vi "AnalogWaveformProbe_I16.vi"(1 "Waveform":waveform(i16)={"t0"=timestamp(0 s since 1904-01-01), "dt"=0.0, "Y"=[]}) -> (0 "Stop if?":bool)   [LabVIEW 2017]
doc: "Displays a graph of the analog data; a table with a time stamp that specifies when the probe received the data, the x value, and the time; and a table that displays the attributes of the waveform data type."
uses:
  <vilib>/Utility/error.llb/ErrWarn.ctl
panel:
  in  "x":string="x"
  in  "t":string="t"
  in  "Tab Control":T1(tab)
  out "Timestamp":timestamp format="%<%X\n%x>T"
  out "Waveform Graph":waveform(i16)(graph) caption="Waveform Graph 2"
  in  "warn icon":T2
  in  "warning msg":string="Table data truncated to\nlimit memory usage."
  out "Start t":timestamp format="%<%X\n%x>T"
  out "Data":string[][](table)
  out "Attributes":variant
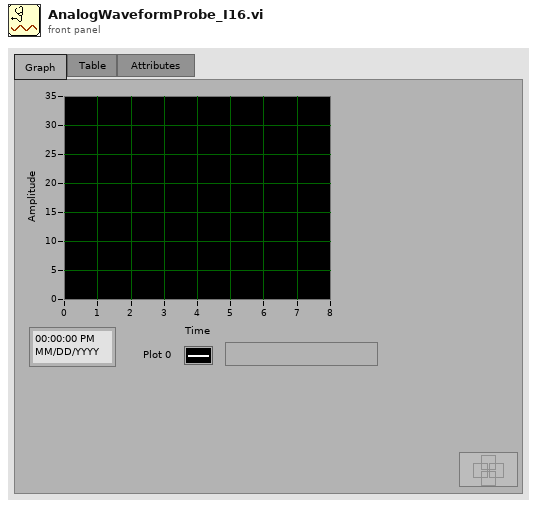
[diagram p1: front panel]
types:
  T1 = enum32{"Graph   ", "Table   ", "Attributes     "}
  T2 = typedef "ErrWarn.ctl" = bool
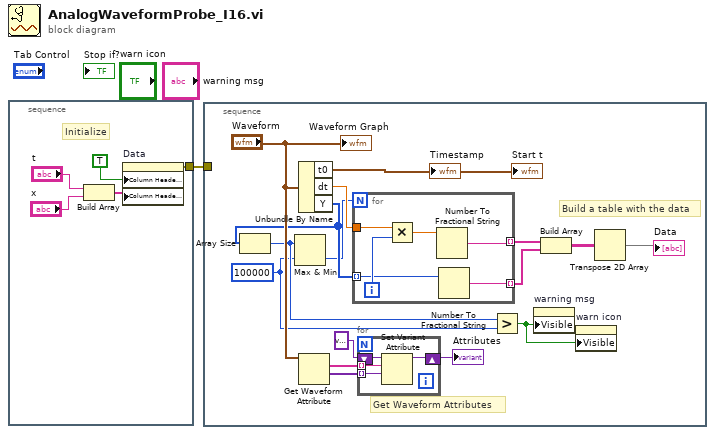
[diagram p0: block diagram]
diagram:
  n1 = stacked-sequence {
    tunnel: [w2] -> w1
    frame #0 {
      # "Initialize"
      n2 = Build Array("t", "x") -> (w4:string[])
      n3 = property on="Data" class="Tbl (strict)"("Column Headers Visible"=TRUE, "Column Header Strings[]"=w4) -> (error out=w2:errorcluster)  [unwired: 2 in, 1 out]
    }
  }
  n4 = stacked-sequence {
    tunnel: w1 -> [_]
    frame #0 {
      w8 = 100000
      # "Get Waveform Attributes"
      # "Build a table with the data"
      n5 = Unbundle By Name("Waveform") -> ("t0"=→"Timestamp" →"Start t":timestamp, "dt"=w22:dbl, "Y"=w11:i16[])
      n6 = Array Size(array=w11) -> (size(s)=w9:i32)
      n7 = Max & Min(x=w9, y=w8) -> (min(x,y)=w10:i32)  [unwired: 1 out]
      n8 = Get Waveform Attribute(7:"Waveform") -> (1:w14:variant[], 2:w15:string[])  [unwired: 3 in, 2 out]
      n9 = for {
        N: w10 -> [_]
        tunnel: [w30] -> w19 mode=indexing
        tunnel: w11 -> [w29] mode=indexing
        tunnel: w22 -> [w32]
        tunnel: [w27] -> w18 mode=indexing
        i -> [w31]
        n10 = Multiply(x=w32, y=w31) -> (x*y=w28:dbl)
        n11 = Number To Fractional String(number=w28) -> (F-format string=w27:string)  [unwired: 3 in]
        n12 = Number To Fractional String(number=w29) -> (F-format string=w30:string)  [unwired: 3 in]
      }
      n13 = for {
        tunnel: w15 -> [w25] mode=indexing
        tunnel: w14 -> [w26] mode=indexing
        shift-right: [w23] -> w12
        shift-left: variant ("variant") -> [w24]
        n14 = Set Variant Attribute(Variant=w24, name=w25, value=w26) -> (Variant out=w23:variant)  [unwired: 1 in, 2 out]
      }
      "Attributes" <- w12
      n15 = Greater?(x=w9, y=w8) -> (0:w7:bool)
      n16 = property on="warning msg" class="Str"("Visible"=w7) -> ()  [unwired: 2 in, 2 out]
      n17 = Build Array(w18, w19) -> (w21:string[][])
      n18 = property on="warn icon" class="Bool"("Visible"=w7) -> ()  [unwired: 2 in, 2 out]
      n19 = Transpose 2D Array(2D array=w21) -> (transposed array=→"Data":string[][])
      "Waveform Graph" <- "Waveform"
    }
  }
